vi "Sub03_PosTxt.vi"(8 "error in (no error)":errorcluster, 10 "String":string, 11 "Application Directory":path) -> (0 "error out":errorcluster, 3 "output cluster":T1, 5 "standard error":string, 7 "standard output":string)   [LabVIEW 2019]
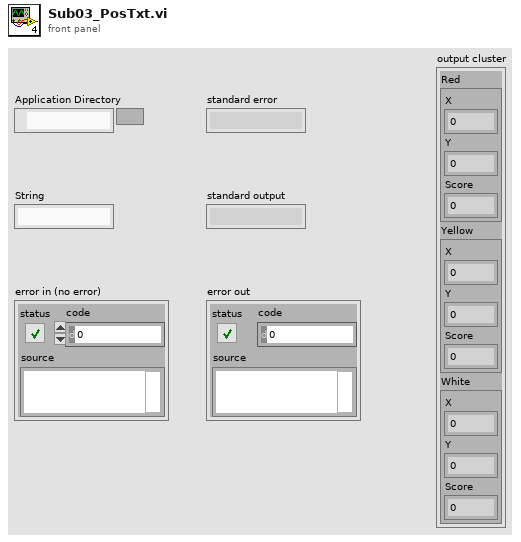
[diagram p1: front panel]
types:
  T1 = cluster{"Red":cluster{"X":u32, "Y":u32, "Score":u32}, "Yellow":cluster{"X":u32, "Y":u32, "Score":u32}, "White":cluster{"X":u32, "Y":u32, "Score":u32}}
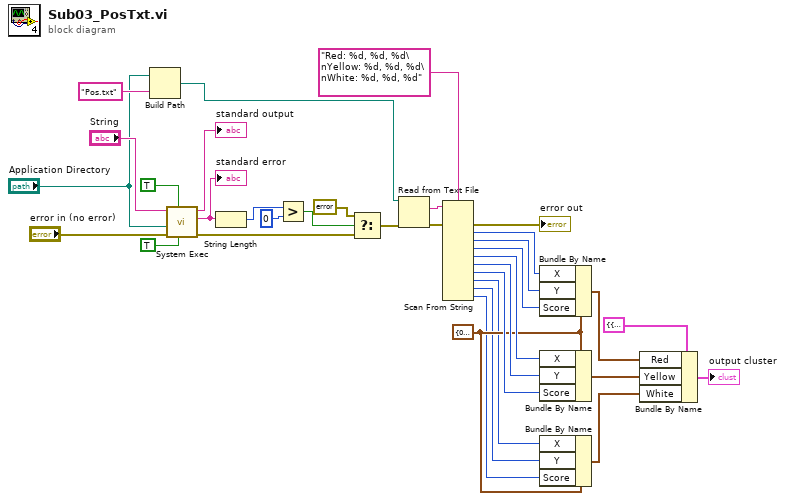
[diagram p0: block diagram]
diagram:
  w9 = cluster{"X":u32, "Y":u32, "Score":u32} {"X"=0, "Y"=0, "Score"=0} ("Cluster")
  n1 = Build Path(base path="Application Directory", name or relative path="Pos.txt") -> (appended path=w20:path)
  n2 = call <vilib>:"System Exec.vi"("run minimized? (F)"=TRUE, "wait until completion? (T)"=TRUE, "error in (no error)"="error in (no error)", "working directory"="Application Directory", "command line"="String") -> ("error out"=w33:errorcluster, "standard error"=w29:string, "standard output"=→"standard output":string)  [unwired: 3 in, 1 out]
  "standard error" <- w29
  n3 = String Length(string=w29) -> (length=w27:i32)
  n4 = Greater?(x=w27, y=0) -> (0:w32:bool)
  n5 = Select(t=errorcluster {"status"=FALSE, "code"=-1, "source"="Pix2Pos execution failed"}, s=w32, f=w33) -> (s? t:f=w21:errorcluster)
  n6 = Read from Text File(file (use dialog)=w20, error in=w21) -> (text=w18:string, error out=w17:errorcluster)  [unwired: 2 in, 2 out]
  n7 = Scan From String(format string="Red: %d, %d, %d\nYellow: %d, %d, %d\nWhite: %d, %d, %d", input string=w18, error in=w17) -> (error out=→"error out":errorcluster, output 1=w15:i32, output 2=w14:i32, output 3=w13:i32, output 4=w12:i32, output 5=w11:i32, output 6=w10:i32, output 7=w8:i32, output 8=w7:i32, output 9=w6:i32)  [unwired: 10 in, 2 out]
  n8 = Bundle By Name(cluster=w9, "X"=w15, "Y"=w14, "Score"=w13) -> (w4:cluster{"X":u32, "Y":u32, "Score":u32})
  n9 = Bundle By Name(cluster=w9, "X"=w12, "Y"=w11, "Score"=w10) -> (w3:cluster{"X":u32, "Y":u32, "Score":u32})
  n10 = Bundle By Name(cluster=w9, "X"=w8, "Y"=w7, "Score"=w6) -> (w2:cluster{"X":u32, "Y":u32, "Score":u32})
  n11 = Bundle By Name(cluster=T1 {"Red"={"X"=0, "Y"=0, "Score"=0}, "Yellow"={"X"=0, "Y"=0, "Score"=0}, "White"={"X"=0, "Y"=0, "Score"=0}} ("output cluster"), "Red"=w4, "Yellow"=w3, "White"=w2) -> (→"output cluster":T1)
